vi "Read File Path Control.vi"(8 "error in (no error)":errorcluster, 11 "Load Measurements Message in":refnum<class "Find Measurements On Disk Message.lvclass">) -> (0 "error out":errorcluster, 2 "Array of Measurement Paths":path[](array[path]), 3 "Load Measurements Message out":refnum<class "Find Measurements On Disk Message.lvclass">)   [LabVIEW 2015, in "Controller Actor.lvlib" / "Find Measurements On Disk Message.lvclass"]
uses:
  Find Measurements On Disk Message.lvclass
  Find Measurements On Disk Message.lvclass/Find Measurements On Disk Message.ctl
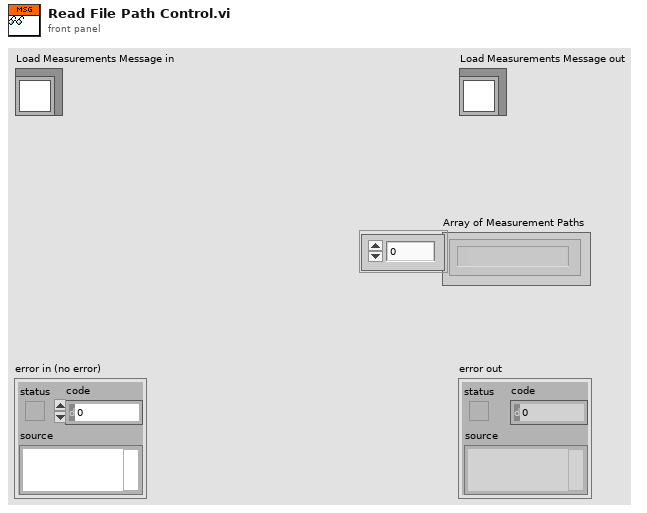
[diagram p1: front panel]
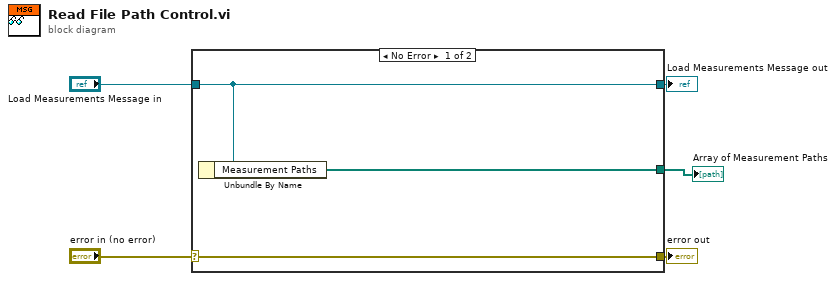
[diagram p0: block diagram]
diagram:
  n1 = case shown="No Error" "error in (no error)" {
    selector: "error in (no error)" -> [w8 w9]
    tunnel: [w8 w9] -> w4
    tunnel: [w7 w10] -> w2
    tunnel: "Load Measurements Message in" -> [w7 w10]
    tunnel: [w6 _] -> w1
    frame No Error {
      n2 = Unbundle By Name(w7) -> ("Measurement Paths"=w6:path[])
    }
    frame Error {
    }
  }
  "error out" <- w4
  "Load Measurements Message out" <- w2
  "Array of Measurement Paths" <- w1
